vi "CAEN_INITIAL (SubVI).vi"(8 "error in (no error)":errorcluster, 11 "Cluster in":T1) -> (0 "error out":errorcluster, 3 "result string":string)   [LabVIEW 2020]
uses:
  Desktop/eTPC/subVIs for MKS/INITIALIZATION PFEIFFER.ctl
  <vilib>/Instr/_visa.llb/VISA Configure Serial Port (Instr).vi
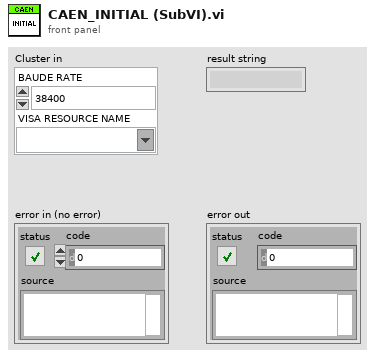
[diagram p1: front panel]
types:
  T1 = typedef "INITIALIZATION PFEIFFER.ctl" = cluster{"BAUDE RATE":enum32{"38400", "19200", "9600", "4800"}, "VISA RESOURCE NAME":refnum<visa-resource-name>}
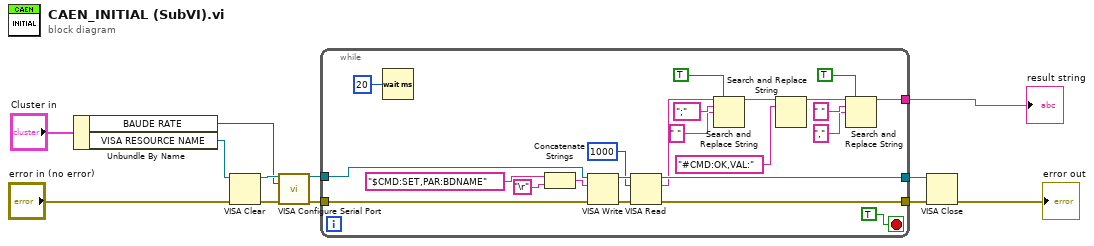
[diagram p0: block diagram]
diagram:
  n1 = Unbundle By Name("Cluster in") -> ("BAUDE RATE"=w3:enum32{"38400", "19200", "9600", "4800"}, "VISA RESOURCE NAME"=w11:refnum<visa-resource-name>)
  n2 = VISA Clear(VISA resource name=w11, error in (no error)="error in (no error)") -> (VISA resource name out=w7:refnum<visa-resource-name>, error out=w8:errorcluster)
  n3 = call-poly "VISA Configure Serial Port"("VISA resource name"=w7, "baud rate (9600)"=w3, "error in (no error)"=w8) -> ("VISA resource name out"=w5:refnum<visa-resource-name>, "error out"=w4:errorcluster)  [unwired: 11 in]
  n4 = while {
    tunnel: w5 -> [w35]
    tunnel: w4 -> [w34]
    tunnel: [w28] -> w2
    tunnel: [w27] -> w1
    tunnel: [w14] -> w12
    stop <- TRUE stop-if-true
    n5 = Wait (ms)(milliseconds to wait=u32 20) -> ()  [unwired: 1 out]
    n6 = Concatenate Strings("$CMD:SET,PAR:BDNAME" ("string"), "\r") -> (w25:string)
    n7 = VISA Write(VISA resource name=w35, write buffer=w25, error in (no error)=w34) -> (VISA resource name out=w30:refnum<visa-resource-name>, error out=w29:errorcluster)  [unwired: 1 out]
    n8 = VISA Read(VISA resource name=w30, byte count=u32 1000, error in (no error)=w29) -> (VISA resource name out=w27:refnum<visa-resource-name>, read buffer=w23:string, error out=w28:errorcluster)  [unwired: 1 out]
    n9 = Search and Replace String(replace all?=TRUE ("replace all? (F)"), input string=w23, search string=";", replace string=" " ("replace string (\"\")")) -> (result string=w18:string)  [unwired: 4 in, 3 out]
    n10 = Search and Replace String(input string=w18, search string="#CMD:OK,VAL:") -> (result string=w13:string)  [unwired: 6 in, 3 out]
    n11 = Search and Replace String(replace all?=TRUE ("replace all? (F)"), input string=w13, search string=" ", replace string="," ("replace string (\"\")")) -> (result string=w14:string)  [unwired: 4 in, 3 out]
  }
  "result string" <- w12
  n12 = VISA Close(VISA resource name=w1, error in (no error)=w2) -> (error out=→"error out":errorcluster)
